vi "Get Data Version.vi"(8 "error in (no error)":errorcluster, 11 "Configuration in":refnum<class "Configuration.lvclass">) -> (0 "error out":errorcluster, 2 "data version":T1, 3 "Configuration out":refnum<class "Configuration.lvclass">)   [LabVIEW 2019, in "DSF Core.lvlib" / "Configuration.lvclass"]
uses:
  Configuration.lvclass
  Typedefs/DSF Version Info.ctl
  DSF Core.lvlib
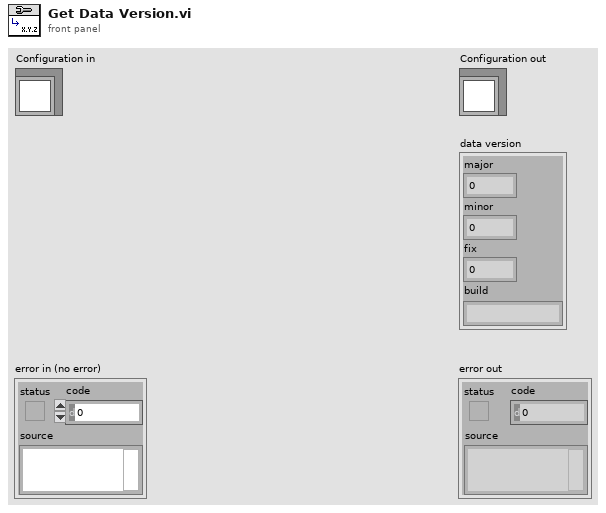
[diagram p1: front panel]
types:
  T1 = typedef "DSF Core.lvlib/DSF Version Info.ctl" = cluster{"major":u32, "minor":u32, "fix":u32, "build":string}
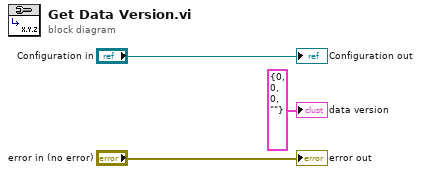
[diagram p0: block diagram]
diagram:
  "error out" <- "error in (no error)"
  "Configuration out" <- "Configuration in"
  "data version" <- T1 {"major"=0, "minor"=0, "fix"=0, "build"=""} ("data version")
